vi "Main Loop.vi"(6 "Stream":T1, 7 "Array":bool[](array[boolean]), 9 "FPGA VI Reference Out":refnum<k20>, 10 "Queue in":refnum<queue>, 11 "Queue in":refnum<queue>) -> ()   [LabVIEW 2015]
uses:
  utilities/GlobalSender.vi
  <vilib>/Utility/error.llb/Error Cluster From Error Code.vi
  <vilib>/rvi/errors/niLvFpgaAdjustHostInterfaceError.vi
  <vilib>/rvi/interface/nirviReadWriteControl/nirviReadWriteControl.xnode
  NiFpgaLv.dll
  <vilib>/rvi/interface/Simulation/niFpgaSimulationCallBeginRW.vi
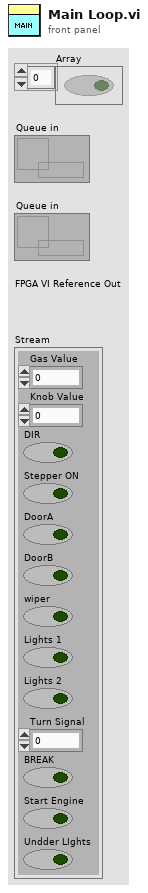
[diagram p1: front panel]
types:
  T1 = cluster{"Gas Value":dbl, "Knob Value":i16, "DIR":bool, "Stepper ON":bool, "DoorA":bool, "DoorB":bool, "wiper":bool, "Lights 1":bool, "Lights 2":bool, "Turn Signal":i8, "BREAK":bool, "Start Engine":bool, "Undder LIghts":bool}
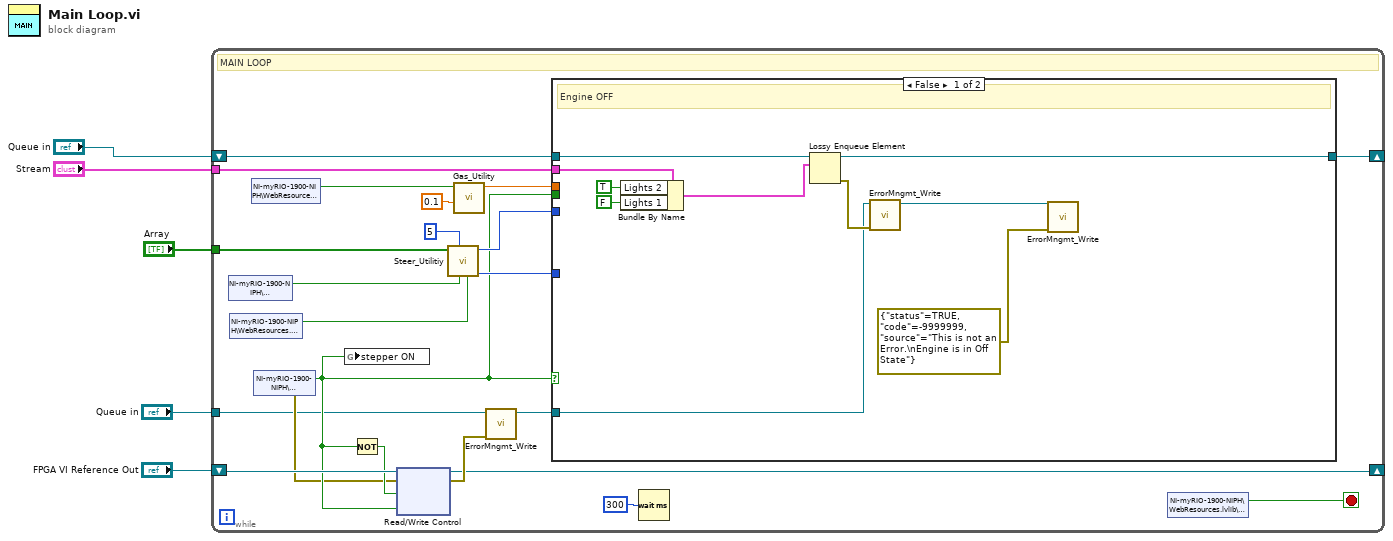
[diagram p0: block diagram]
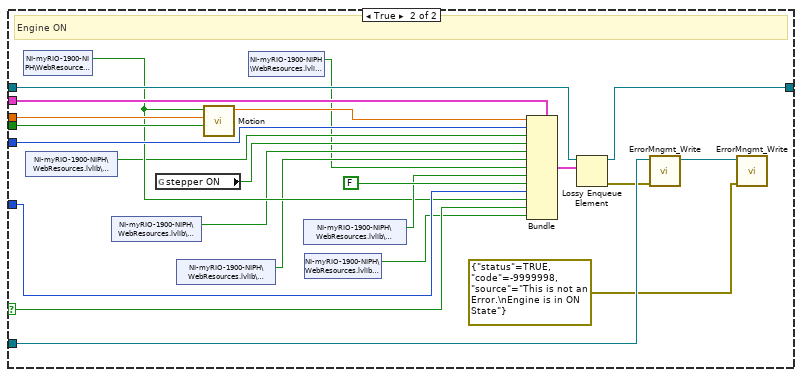
[diagram p2: hidden frame]
diagram:
  n1 = while {
    tunnel: "Stream" -> [w26]
    tunnel: "Array" -> [w22]
    tunnel: "Queue in" -> [w13]
    shift-right: [w11] -> _
    shift-left: "Queue in" -> [w27]
    shift-right: [w10] -> _
    shift-left: "FPGA VI Reference Out" -> [w18]
    stop <- w9 stop-if-true
    # "MAIN LOOP"
    n2 = shared-variable "NI-myRIO-1900-NIPH\\WebResources.lvlib\\Left"() -> (w8:bool)  [unwired: 1 in, 1 out]
    n3 = shared-variable "NI-myRIO-1900-NIPH\\WebResources.lvlib\\Right"() -> (w7:bool)  [unwired: 1 in, 1 out]
    n4 = shared-variable "NI-myRIO-1900-NIPH\\WebResources.lvlib\\Start"() -> (w6:bool)  [unwired: 1 in, 1 out]
    n5 = shared-variable "NI-myRIO-1900-NIPH\\WebResources.lvlib\\Key"() -> (w16:bool, error out=w15:errorcluster)  [unwired: 1 in]
    n6 = global write "GlobalSender.vi" "stepper ON"(w16) -> ()
    n7 = Not(x=w16) -> (.not. x?=w17:bool)
    n8 = xnode "Read/Write Control"("FPGA VI Reference In"=w18, "error in"=w15, "LED0"=w17, "LED1"=w16) -> ("FPGA VI Reference Out"=w10:refnum<k20>, "error out"=w14:errorcluster)
    n9 = call "Steer_Utilitiy.vi"("right"=w7, "left"=w8, "increment"=i16 5, "Array"=w22) -> ("Turn Signal"=w19:i8, "steer"=w24:i16)  [unwired: 6 in]
    n10 = call "Gas_Utility.vi"("increment"=0.1, "GAS"=w6) -> ("coerced"=w20:dbl)  [unwired: 9 in]
    n11 = call "ErrorMngmt_Write.vi"("error in (no error)"=w14, "Queue in"=w13) -> ("Queue out"=w12:refnum<queue>)  [unwired: 8 in, 1 out]
    n12 = case shown="False" w16 {
      selector: w16 -> [_ w54]
      tunnel: w27 -> [w37 w60]
      tunnel: w26 -> [w36 w59]
      tunnel: w20 -> [_ w57]
      tunnel: w24 -> [_ w50]
      tunnel: w16 -> [_ w53]
      tunnel: w19 -> [_ w51]
      tunnel: w12 -> [w32 w49]
      tunnel: [w29 w45] -> w11
      frame False {
        # "Engine OFF"
        n13 = Bundle By Name(cluster=w36, "Lights 2"=TRUE, "Lights 1"=FALSE) -> (w34:T1)
        n14 = Lossy Enqueue Element(queue=w37, element=w34) -> (queue out=w29:refnum<queue>, error out=w33:errorcluster)  [unwired: 1 in, 2 out]
        n15 = call "ErrorMngmt_Write.vi"("error in (no error)"=w33, "Queue in"=w32) -> ("Queue out"=w30:refnum<queue>)  [unwired: 8 in, 1 out]
        n16 = call "ErrorMngmt_Write.vi"("error in (no error)"=errorcluster {"status"=TRUE, "code"=-9999999, "source"="This is not an Error.\nEngine is in Off State"}, "Queue in"=w30) -> ()  [unwired: 8 in, 2 out]
      }
      frame True {
        # "Engine ON"
        n17 = shared-variable "NI-myRIO-1900-NIPH\\WebResources.lvlib\\Stop"() -> (w43:bool)  [unwired: 1 in, 1 out]
        n18 = shared-variable "NI-myRIO-1900-NIPH\\WebResources.lvlib\\Direction"() -> (w40:bool)  [unwired: 1 in, 1 out]
        n19 = shared-variable "NI-myRIO-1900-NIPH\\WebResources.lvlib\\LeftDoor"() -> (w41:bool)  [unwired: 1 in, 1 out]
        n20 = global read "GlobalSender.vi" "stepper ON"() -> (w52:bool)
        n21 = shared-variable "NI-myRIO-1900-NIPH\\WebResources.lvlib\\RightDoor"() -> (w42:bool)  [unwired: 1 in, 1 out]
        n22 = call "Motion.vi"("engine start"=w53, "coerced"=w57, "BRAKES"=w43) -> ("upper limit"=w56:dbl)  [unwired: 8 in]
        n23 = shared-variable "NI-myRIO-1900-NIPH\\WebResources.lvlib\\Wiper"() -> (w39:bool)  [unwired: 1 in, 1 out]
        n24 = shared-variable "NI-myRIO-1900-NIPH\\WebResources.lvlib\\HeadLights"() -> (w44:bool)  [unwired: 1 in, 1 out]
        n25 = shared-variable "NI-myRIO-1900-NIPH\\WebResources.lvlib\\Under"() -> (w38:bool)  [unwired: 1 in, 1 out]
        n26 = Bundle(cluster=w59, "Gas Value"=w56, "Knob Value"=w50, "DIR"=w40, "Stepper ON"=w52, "DoorA"=w41, "DoorB"=w42, "wiper"=w39, "Lights 1"=w44, "Lights 2"=FALSE, "Turn Signal"=w51, "BREAK"=w43, "Start Engine"=w54, "Undder LIghts"=w38) -> (w58:T1)
        n27 = Lossy Enqueue Element(queue=w60, element=w58) -> (queue out=w45:refnum<queue>, error out=w48:errorcluster)  [unwired: 1 in, 2 out]
        n28 = call "ErrorMngmt_Write.vi"("error in (no error)"=w48, "Queue in"=w49) -> ("Queue out"=w47:refnum<queue>)  [unwired: 8 in, 1 out]
        n29 = call "ErrorMngmt_Write.vi"("error in (no error)"=errorcluster {"status"=TRUE, "code"=-9999998, "source"="This is not an Error.\nEngine is in ON State"}, "Queue in"=w47) -> ()  [unwired: 8 in, 2 out]
      }
    }
    n30 = Wait (ms)(milliseconds to wait=u32 300) -> ()  [unwired: 1 out]
    n31 = shared-variable "NI-myRIO-1900-NIPH\\WebResources.lvlib\\Engine"() -> (w9:bool)  [unwired: 1 in, 1 out]
  }
